vi "Dialog.Error Message.vi"(1 "error in":errorcluster) -> (0 "Selection":enum16{"Exit", "Reset", "Ignore"}(ring)=enum."Reset")   [LabVIEW 2018]
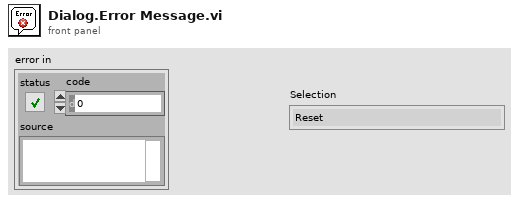
[diagram p1: front panel]
types:
  T1 = enum16{"Left Button", "Center Button", "Right Button", "Window Close"}
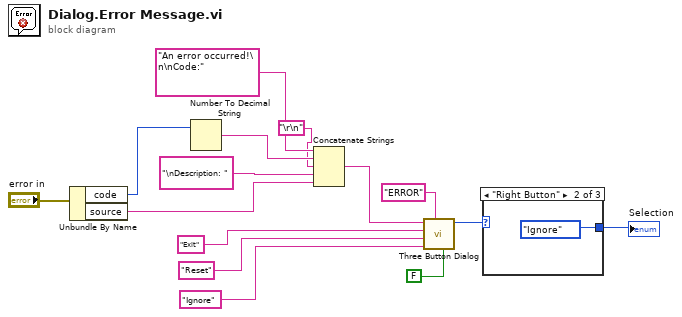
[diagram p0: block diagram]
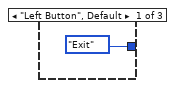
[diagram p2: hidden frame]
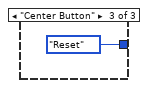
[diagram p3: hidden frame]
diagram:
  n1 = Unbundle By Name("error in") -> ("code"=w9:i32, "source"=w10:string)
  n2 = Number To Decimal String(number=w9) -> (decimal integer string=w13:string)  [unwired: 1 in]
  n3 = Concatenate Strings("An error occurred!\n\nCode:", w13, "\r\n", "\nDescription: ", w10) -> (w8:string)
  n4 = call <vilib>:"Three Button Dialog.vi"("Allow user to close window? (TRUE)"=FALSE, "Window Title (\"\")"="ERROR" ("Window Title (\"\")"), "Right Button Text (\"Cancel\")"="Ignore", "Center Button Text (\"No\")"="Reset", "Left Button Text (\"Yes\")"="Exit", "message"=w8) -> ("Which Button?"=w2:T1)  [unwired: 5 in]
  n5 = case shown="\"Right Button\"" w2 {
    tunnel: [enum16{"Exit", "Reset", "Ignore"}."Exit" ("Selection") enum16{"Exit", "Reset", "Ignore"}."Ignore" ("Selection") enum16{"Exit", "Reset", "Ignore"}."Reset" ("Selection")] -> w1
    frame "Left Button", Default {
    }
    frame "Right Button" {
    }
    frame "Center Button" {
    }
  }
  "Selection" <- w1
